vi "Servo home&Fault.vi"(8 "error in (no error)":errorcluster, 11 "Queue in":refnum<queue>) -> (0 "error out":errorcluster, 1 "Servo Fault":bool, 2 "Home":bool, 3 "Queue out":refnum<queue>)   [LabVIEW 2015]
uses:
  Testing/Test  enqueue/AutoTest seq.ctl
  Galobal variable_TI.vi
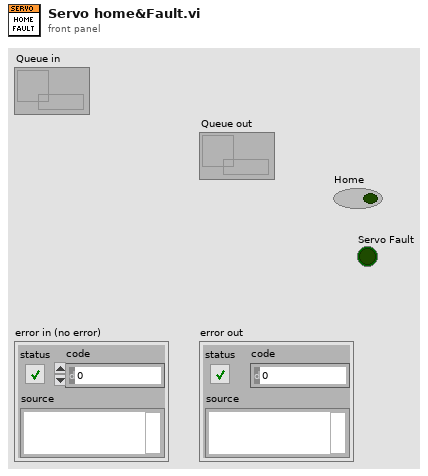
[diagram p1: front panel]
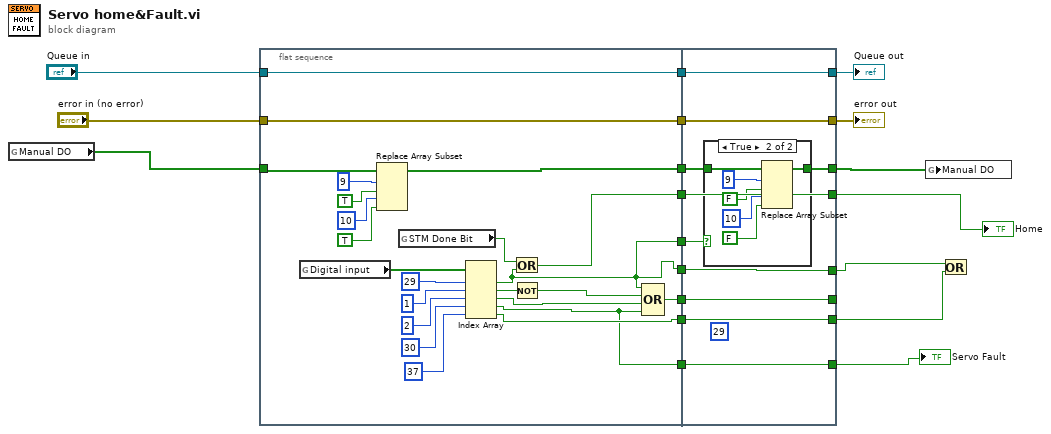
[diagram p0: block diagram]
diagram:
  n1 = global read "Galobal variable_TI.vi" "Manual DO"() -> (w9:bool[])
  n2 = flat-sequence {
    tunnel: "Queue in" -> [w40]
    tunnel: "error in (no error)" -> [w39]
    tunnel: [w40] -> w19
    tunnel: [w39] -> w18
    tunnel: [w33] -> w17
    tunnel: [w22] -> w16
    tunnel: w9 -> [w29]
    tunnel: [w22] -> w15
    tunnel: [w25] -> w10
    tunnel: [w23] -> w6
    tunnel: [w21] -> w5
    tunnel: [w20] -> w2
    tunnel: [w51] -> w14
    tunnel: [w52] -> w13
    tunnel: w19 -> [w52]
    tunnel: w18 -> [w51]
    tunnel: w17 -> [w50]
    tunnel: [w49] -> w8
    tunnel: w16 -> [w48]
    tunnel: [w47] -> w4
    tunnel: w15 -> [w47]
    tunnel: [w46] -> _
    tunnel: w10 -> [w46]
    tunnel: [w45] -> w7
    tunnel: w6 -> [w45]
    tunnel: [w44] -> w1
    tunnel: w5 -> [w44]
    tunnel: [w43] -> w3
    tunnel: w2 -> [w43]
    frame #0 {
      n3 = global read "Galobal variable_TI.vi" "Digital input"() -> (w38:bool[])
      n4 = Replace Array Subset(array=w29, new element #1=TRUE ("new element/subarray"), index #1=9 ("index"), new element #2=TRUE ("new element/subarray"), index #2=10 ("index")) -> (w33:bool[])
      n5 = global read "Galobal variable_TI.vi" "STM Done Bit"() -> (w41:bool)
      n6 = Index Array(array=w38, index #1=29 ("index"), index #2=1 ("index"), index #3=2 ("index"), index #4=30 ("index"), index #5=37 ("index")) -> (element #1=w22:bool, element #2=w31:bool, element #3=w27:bool, element #4=w21:bool, element #5=w23:bool)
      n7 = Or(x=w41, y=w22) -> (x .or. y?=w20:bool)
      n8 = Not(x=w31) -> (.not. x?=w30:bool)
      n9 = Compound Arithmetic op=OR(w22, w30, w27, w21) -> (w25:bool)
    }
    frame #1 {
      (unwired) 29 ("index")
      n10 = case shown="True" w48 {
        tunnel: w50 -> [w53 w55]
        tunnel: [w53 w54] -> w49
        frame False {
        }
        frame True {
          n11 = Replace Array Subset(array=w55, new element #1=FALSE ("new element/subarray"), index #1=9 ("index"), new element #2=FALSE ("new element/subarray"), index #2=10 ("index")) -> (w54:bool[])
        }
      }
    }
  }
  n12 = global write "Galobal variable_TI.vi" "Manual DO"(w8) -> ()
  n13 = Or(x=w4, y=w7) -> ()  [unwired: 1 out]
  "Home" <- w3
  "error out" <- w14
  "Queue out" <- w13
  "Servo Fault" <- w1
